vi "197-Caller flow of async message.vi"() -> ()   [LabVIEW 2017]
uses:
  user.lib/_NEVSTOP/Communicable State Machine(CSM)/Communicable State Machine.lvlib
panel:
  out "Waveform Chart":i32(graph)
  out "Response":string="DoA"
  out "#Flushed":cluster{i32, i32}
  in  "flush":bool
  out "#msg to be processed":i32
  out "Diff Timer(s)":dbl format="%.6f"
  out "error IO":errorcluster
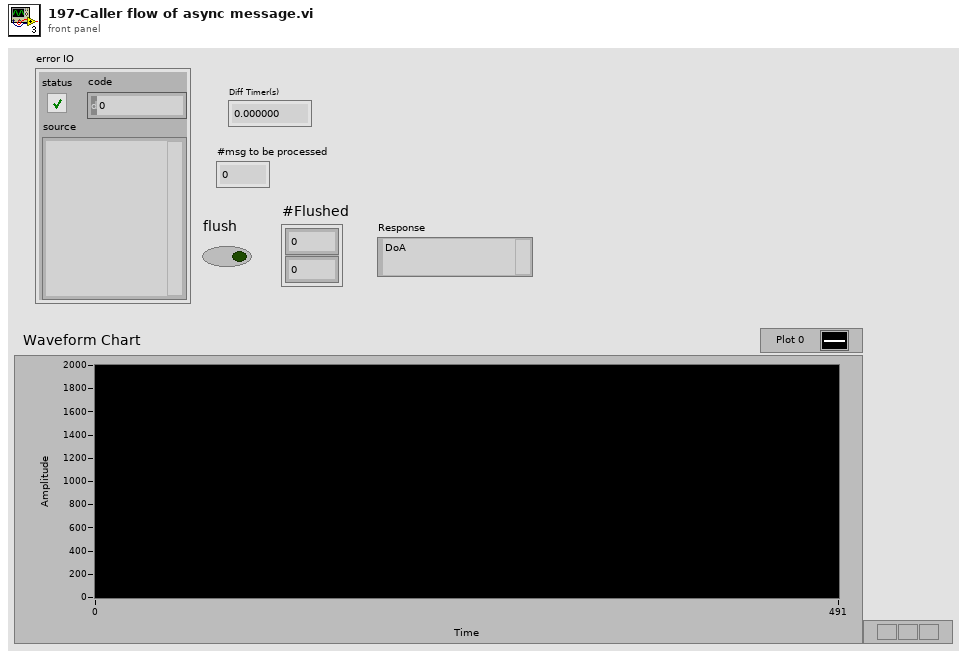
[diagram p1: front panel]
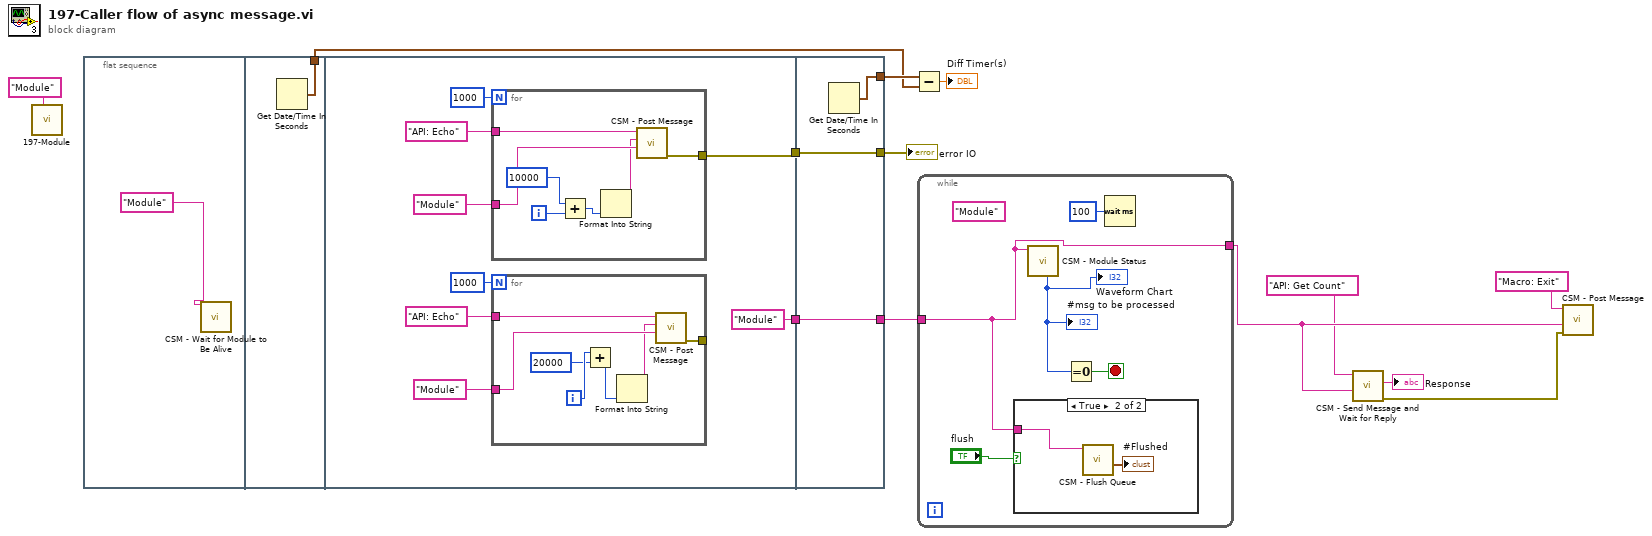
[diagram p0: block diagram]
diagram:
  n1 = call "197-Module.vi"("Name(\"\" to use uuid)"="Module" ("Name(\"\" to use uuid)")) -> ()  [unwired: 11 in]
  n2 = flat-sequence {
    tunnel: [w15] -> w7
    tunnel: [w19] -> w11
    tunnel: ["Module" ("Name(\"\" to use uuid)")] -> w10
    tunnel: [w39] -> w5
    tunnel: [w40] -> w12
    tunnel: w11 -> [w40]
    tunnel: w10 -> [w39]
    tunnel: [w38] -> w9
    frame #0 {
      n3 = call "CSM - Wait for Module to Be Alive.vi"("CSM Name"="Module" ("Name(\"\" to use uuid)")) -> ()  [unwired: 12 in, 3 out]
    }
    frame #1 {
      n4 = Get Date/Time In Seconds() -> (seconds since 1Jan1904=w15:timestamp)
    }
    frame #2 {
      n5 = for {
        N: 1000 -> [_]
        tunnel: "API: Echo" ("State") -> [w37]
        tunnel: "Module" ("Name(\"\" to use uuid)") -> [w36]
        tunnel: [w35] -> w19
        i -> [w33]
        n6 = Add(x=10000, y=w33) -> (x+y=w32:i32)
        n7 = Format Into String(w32) -> (resulting string=w34:string)  [unwired: 3 in, 1 out]
        n8 = call "CSM - Post Message.vi"("Target Module"=w36, "Arguments (\"\")"=w34, "State"=w37) -> ("error out"=w35:errorcluster)  [unwired: 8 in]
      }
      n9 = for {
        N: 1000 -> [_]
        tunnel: "API: Echo" ("State") -> [w30]
        tunnel: "Module" ("Name(\"\" to use uuid)") -> [w29]
        tunnel: [w28] -> _
        i -> [w27]
        n10 = Add(x=w27, y=20000 ("x")) -> (x+y=w25:i32)
        n11 = Format Into String(w25) -> (resulting string=w26:string)  [unwired: 3 in, 1 out]
        n12 = call "CSM - Post Message.vi"("Target Module"=w29, "Arguments (\"\")"=w26, "State"=w30) -> ("error out"=w28:errorcluster)  [unwired: 8 in]
      }
    }
    frame #3 {
      n13 = Get Date/Time In Seconds() -> (seconds since 1Jan1904=w38:timestamp)
    }
  }
  n14 = Subtract(x=w9, y=w7) -> (x-y=→"Diff Timer(s)":dbl)
  n15 = while {
    tunnel: w5 -> [w42]
    tunnel: [w42] -> w4
    stop <- w45 stop-if-true
    (unwired) "Module" ("Name(\"\" to use uuid)")
    n16 = case shown="True" "flush" {
      tunnel: w42 -> [_ w47]
      frame False {
      }
      frame True {
        n17 = call "CSM - Flush Queue.vi"("CSM Name"=w47) -> ("#Flushed"=→"#Flushed":cluster{i32, i32})  [unwired: 8 in, 2 out]
      }
    }
    n18 = call "CSM - Module Status.vi"("CSM Name"=w42) -> ("#Elements In Queue"=w41:i32)  [unwired: 6 in, 4 out]
    "#msg to be processed" <- w41
    "Waveform Chart" <- w41
    n19 = Equal To 0?(x=w41) -> (x = 0?=w45:bool)
    n20 = Wait (ms)(milliseconds to wait=u32 100) -> ()  [unwired: 1 out]
  }
  n21 = call "CSM - Send Message and Wait for Reply.vi"("Target Module"=w4, "State"="API: Get Count") -> ("error out"=w3:errorcluster, "Response"=→"Response":string)  [unwired: 7 in, 1 out]
  n22 = call "CSM - Post Message.vi"("Error In (No Error)"=w3, "Target Module"=w4, "State"="Macro: Exit") -> ()  [unwired: 8 in, 1 out]
  "error IO" <- w12
